vi "svacg_LimitTest Create Input Frequency Cluster based Limit.vi"(0 "signal in":cluster{"f0":dbl, "df":dbl, "spectrum":dbl[]}={"f0"=0.0, "df"=1.0, "spectrum"=[]} {"spectrum" format="%.2p"; "df" format="%0.2p"; "f0" format="%0.2p"}, 1 "open interval? (T)":bool=TRUE, 5 "df":dbl=1.0 format="%.2p", 7 "f0":dbl, 9 "interpolation mode":u16(ring)=1 items=["coerce", "linear", "spline", "FIR filter"], 11 "error in":errorcluster, 12 "FIR filter specifications":T2={"alias rejection (dB)"=120.0, "normalized bandwidth"=0.4536} {"normalized bandwidth" format="%.4f"; "alias rejection (dB)" format="%.2f"}, 13 "Protection limits":T1={"Max oversampling ratio"=1024.0, "Max # output samples"=2097150}) -> (4 "upper limit":cluster{"f0":dbl, "df":dbl, "data":dbl[]}={"f0"=0.0, "df"=1.0, "data"=[]} {"data" format="%.2p"; "df" format="%.2p"; "f0" format="%.2p"}, 10 "used f0":dbl format="%.2p", 14 "f0 adjusted warning":bool, 15 "error out":errorcluster)   [LabVIEW 2017]
uses:
  <vilib>/measure/NI_MAPro.lvlib
panel:
  # "open"
  # "closed"
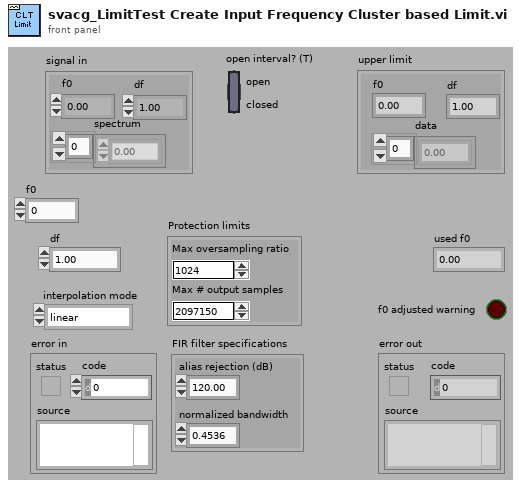
[diagram p1: front panel]
types:
  T1 = cluster{"Max oversampling ratio":dbl, "Max # output samples":i32}
  T2 = cluster{"alias rejection (dB)":dbl, "normalized bandwidth":dbl}
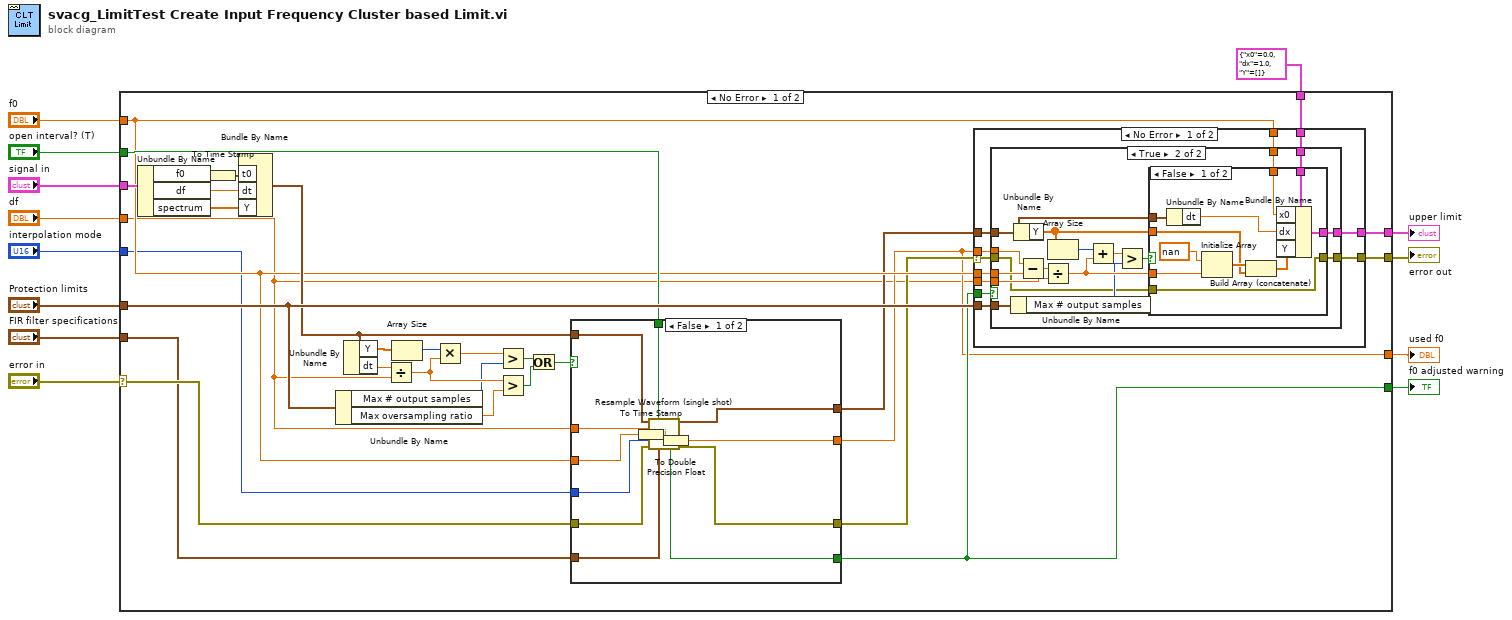
[diagram p0: block diagram]
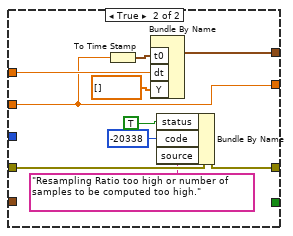
[diagram p2: hidden frame]
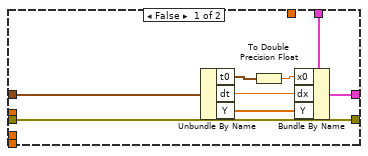
[diagram p3: hidden frame]
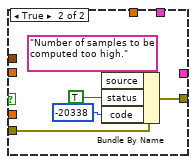
[diagram p4: hidden frame]
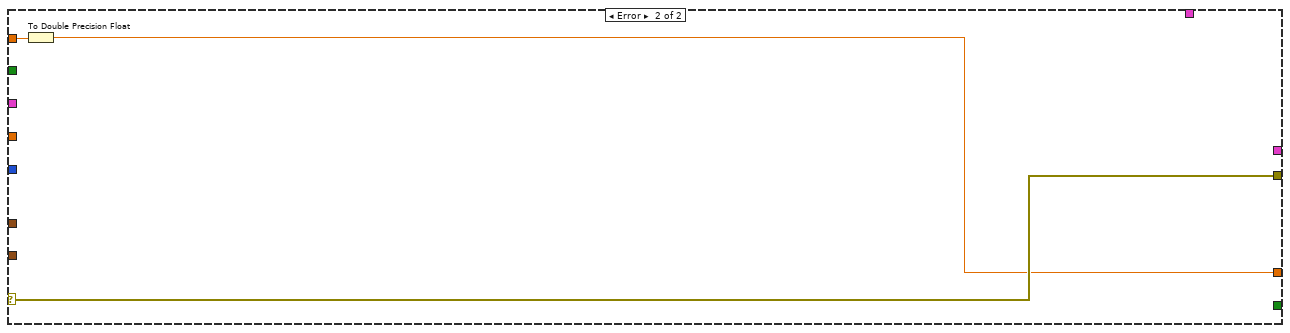
[diagram p6: hidden frame]
diagram:
  n1 = case shown="No Error" "error in" {
    selector: "error in" -> [w20 w122]
    tunnel: [w42 w122] -> w12
    tunnel: "signal in" -> [w36 _]
    tunnel: "df" -> [w14 _]
    tunnel: "f0" -> [w22 w121]
    tunnel: "Protection limits" -> [w25 _]
    tunnel: [w43 _] -> w2
    tunnel: "FIR filter specifications" -> [w19 _]
    tunnel: "interpolation mode" -> [w21 _]
    tunnel: "open interval? (T)" -> [w24 _]
    tunnel: [w16 w120] -> w4
    tunnel: [w18 _] -> w3
    tunnel: cluster{"x0":dbl, "dx":dbl, "Y":dbl[]} {"x0"=0.0, "dx"=1.0, "Y"=[]} ("upper limit") -> [w41 _]
    frame No Error {
      n2 = Unbundle By Name(w36) -> ("f0"=w38:dbl, "df"=w39:dbl, "spectrum"=w40:dbl[])
      n3 = To Time Stamp(1:w38) -> (0:w37:timestamp)
      n4 = Bundle By Name("t0"=w37, "dt"=w39, "Y"=w40) -> (w23:waveform(dbl))  [unwired: 1 in]
      n5 = Unbundle By Name(w25) -> ("Max # output samples"=w26:i32, "Max oversampling ratio"=w27:dbl)
      n6 = Unbundle By Name(w23) -> ("Y"=w34:dbl[], "dt"=w35:dbl)
      n7 = Divide(x=w35, y=w14) -> (x/y=w32:dbl)
      n8 = Array Size(array=w34) -> (size(s)=w33:i32)
      n9 = Multiply(x=w33, y=w32) -> (x*y=w31:dbl)
      n10 = Greater?(x=w31, y=w26) -> (0:w30:bool)
      n11 = Greater?(x=w32, y=w27) -> (0:w29:bool)
      n12 = Or(x=w30, y=w29) -> (x .or. y?=w28:bool)
      n13 = case shown="False" w28 {
        tunnel: [w56 w63] -> w15
        tunnel: w20 -> [w55 w61]
        tunnel: [w54 w60] -> w17
        tunnel: w19 -> [w53 _]
        tunnel: w21 -> [w52 _]
        tunnel: w22 -> [w51 w62]
        tunnel: [w50 w62] -> w16
        tunnel: [w49 _] -> w18
        tunnel: w24 -> [w48 _]
        tunnel: w23 -> [w47 _]
        tunnel: w14 -> [w46 w65]
        frame False {
          n14 = To Time Stamp(1:w51) -> (0:w45:timestamp)
          n15 = call <vilib>:"Resample Waveform (single shot).vi"("waveform in"=w47, "open interval? (F)"=w48, "dt"=w46, "t0"=w45, "interpolation mode"=w52, "error in (no error)"=w55, "FIR filter specifications"=w53) -> ("resampled waveform out"=w56:waveform(dbl), "used t0"=w44:timestamp, "t0 adjusted warning"=w49:bool, "error out"=w54:errorcluster)  [unwired: 5 in]
          n16 = To Double Precision Float(number=w44) -> (double precision float=w50:dbl)
        }
        frame True {
          n17 = To Time Stamp(1:w62) -> (0:w66:timestamp)
          n18 = Bundle By Name("t0"=w66, "dt"=w65, "Y"=dbl[] []) -> (w63:waveform(dbl))  [unwired: 1 in]
          n19 = Bundle By Name(cluster=w61, "status"=TRUE, "code"=-20338, "source"="Resampling Ratio too high or number of samples to be computed too high.") -> (w60:errorcluster)
        }
      }
      n20 = case shown="No Error" w17 {
        selector: w17 -> [w68 w119]
        tunnel: w15 -> [w77 _]
        tunnel: w16 -> [w76 _]
        tunnel: w14 -> [w75 _]
        tunnel: w22 -> [w74 _]
        tunnel: w22 -> [w73 _]
        tunnel: w18 -> [w72 _]
        tunnel: [w71 _] -> w43
        tunnel: [w69 w119] -> w42
        tunnel: w25 -> [w70 _]
        tunnel: w41 -> [w67 _]
        frame No Error {
          n21 = case shown="True" w72 {
            tunnel: [w80 w100] -> w71
            tunnel: w77 -> [w81 w99]
            tunnel: w76 -> [_ w96]
            tunnel: w74 -> [_ w97]
            tunnel: w75 -> [_ w101]
            tunnel: w73 -> [_ w98]
            tunnel: w70 -> [_ w91]
            tunnel: [w85 w88] -> w69
            tunnel: w68 -> [w85 w87]
            tunnel: w67 -> [w79 w86]
            frame False {
              n22 = Unbundle By Name(w81) -> ("t0"=w83:timestamp, "dt"=w78:dbl, "Y"=w82:dbl[])
              n23 = To Double Precision Float(number=w83) -> (double precision float=w84:dbl)
              n24 = Bundle By Name(cluster=w79, "x0"=w84, "dx"=w78, "Y"=w82) -> (w80:cluster{"x0":dbl, "dx":dbl, "Y":dbl[]})
            }
            frame True {
              n25 = Unbundle By Name(w91) -> ("Max # output samples"=w90:i32)
              n26 = Unbundle By Name(w99) -> ("Y"=w95:dbl[])
              n27 = Subtract(x=w96, y=w97) -> (x-y=w102:dbl)
              n28 = Divide(x=w102, y=w101) -> (x/y=w93:dbl)
              n29 = Array Size(array=w95) -> (size(s)=w94:i32)
              n30 = Add(x=w94, y=w93) -> (x+y=w92:dbl)
              n31 = Greater?(x=w92, y=w90) -> (0:w89:bool)
              n32 = case shown="False" w89 {
                tunnel: [w108 _] -> w100
                tunnel: w99 -> [w104 _]
                tunnel: w98 -> [w107 _]
                tunnel: w95 -> [w111 _]
                tunnel: w93 -> [w110 _]
                tunnel: [w109 w115] -> w88
                tunnel: w87 -> [w109 w116]
                tunnel: w86 -> [w105 _]
                frame False {
                  n33 = Unbundle By Name(w104) -> ("dt"=w103:dbl)
                  n34 = Initialize Array(nan, w110) -> (w112:dbl[])
                  n35 = Build Array (concatenate)(w112, w111) -> (w106:dbl[])
                  n36 = Bundle By Name(cluster=w105, "x0"=w107, "dx"=w103, "Y"=w106) -> (w108:cluster{"x0":dbl, "dx":dbl, "Y":dbl[]})
                }
                frame True {
                  n37 = Bundle By Name(cluster=w116, "source"="Number of samples to be computed too high.", "status"=TRUE, "code"=-20338) -> (w115:errorcluster)
                }
              }
            }
          }
        }
        frame Error {
        }
      }
    }
    frame Error {
      n38 = To Double Precision Float(number=w121) -> (double precision float=w120:dbl)
    }
  }
  "upper limit" <- w2
  "error out" <- w12
  "f0 adjusted warning" <- w3
  "used f0" <- w4
